vi "fake_80kHz_trigger.vi"(0 "Counter in":u16) -> (1 "trigger":bool, 2 "Counter out":u16)   [LabVIEW 2010]
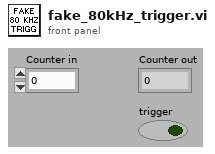
[diagram p1: front panel]
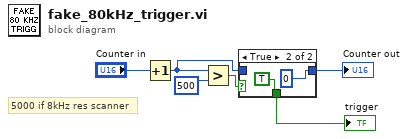
[diagram p0: block diagram]
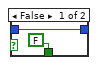
[diagram p2: hidden frame]
diagram:
  # "5000 if 8kHz res scanner"
  n1 = Increment(x="Counter in") -> (x+1=w6:u16)
  n2 = Greater?(x=w6, y=u16 500 ("res scanner freq (in loop time)")) -> (0:w1:bool)
  n3 = case shown="True" w1 {
    tunnel: [w8 u16 0] -> w4
    tunnel: [FALSE ("OFF") TRUE ("OFF")] -> w5
    tunnel: w6 -> [w8 _]
    frame False {
    }
    frame True {
    }
  }
  "trigger" <- w5
  "Counter out" <- w4
